vi "traces_free_find.vi"(0 "Thorlabs_OSA_64 in":refnum<class "OSA.lvclass">, 2 "idx start":i32, 4 "traces idx":cluster{"idx":u32}[](array[cluster]), 5 "error in (no error)":errorcluster, 6 "buffer size":i32, 7 "allocate X-array":bool) -> (14 "Thorlabs_OSA_64 out":refnum<class "OSA.lvclass">, 16 "idx found":i32, 18 "traces idx out":cluster{"idx":u32}[](array[cluster]), 19 "error out":errorcluster)   [LabVIEW 2010, in "OSA.lvclass"]
uses:
  OSA.lvclass
  FTSLib.dll
  OSA20X_misc.lvlib
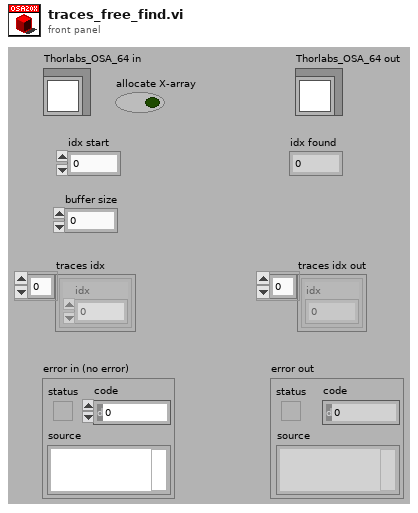
[diagram p1: front panel]
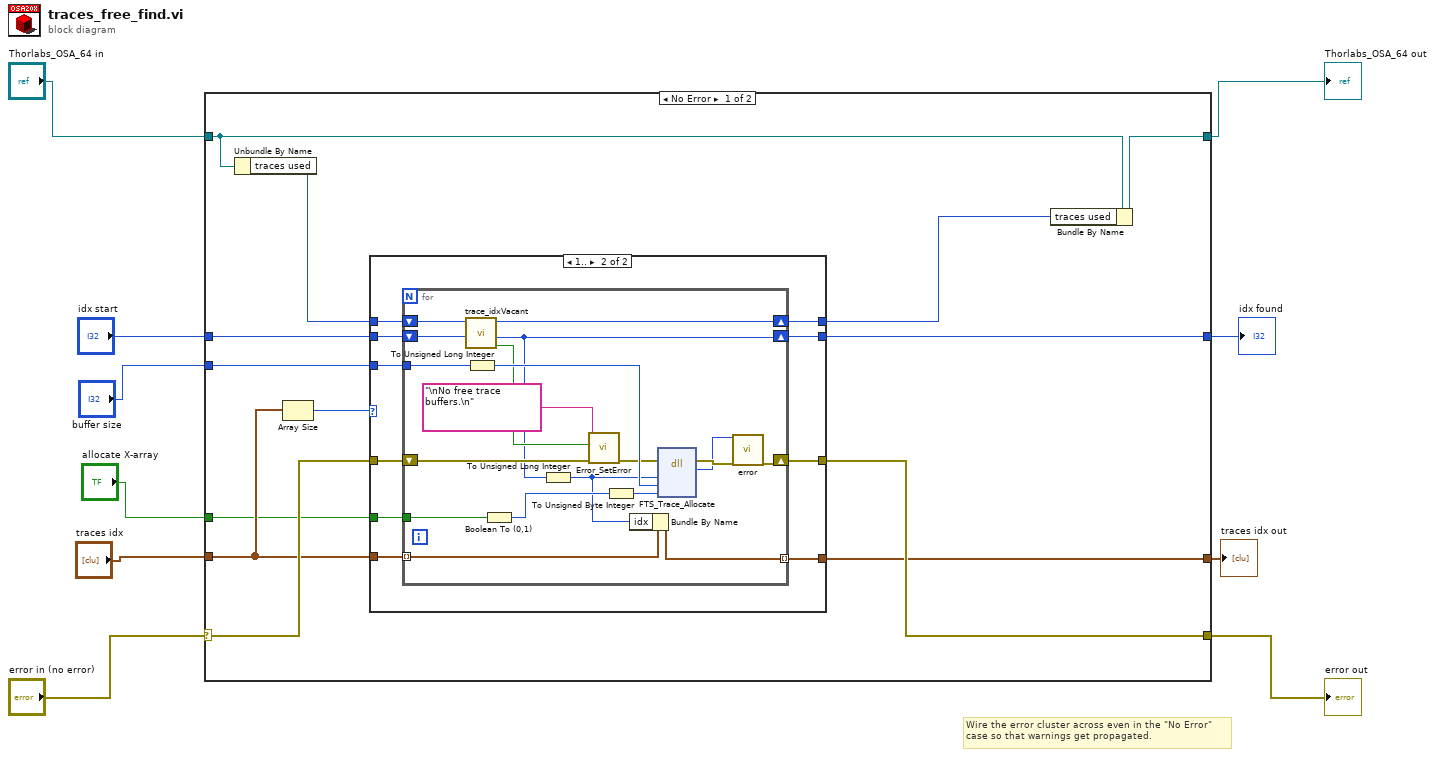
[diagram p0: block diagram]
diagram:
  # "Wire the error cluster across even in the \"No Error\"\ncase so that warnings get propagated."
  n1 = case shown="No Error" "error in (no error)" {
    selector: "error in (no error)" -> [w18 w60]
    tunnel: [w17 w60] -> w5
    tunnel: "idx start" -> [w20 w57]
    tunnel: [w19 w57] -> w9
    tunnel: "traces idx" -> [w16 w58]
    tunnel: [w15 w58] -> w7
    tunnel: "Thorlabs_OSA_64 in" -> [w14 w59]
    tunnel: [w13 w59] -> w3
    tunnel: "buffer size" -> [w12 _]
    tunnel: "allocate X-array" -> [w11 _]
    frame No Error {
      n2 = Unbundle By Name(w14) -> ("traces used"=w22:u64)
      n3 = Array Size(array=w16) -> (size(s)=w23:i32)
      n4 = case shown="1.." w23 {
        tunnel: w18 -> [w27 w37]
        tunnel: w12 -> [_ w36]
        tunnel: [w27 w35] -> w17
        tunnel: w16 -> [w26 w34]
        tunnel: [w26 w33] -> w15
        tunnel: w22 -> [w25 w32]
        tunnel: w20 -> [w24 w31]
        tunnel: [w25 w30] -> w21
        tunnel: [w24 w29] -> w19
        tunnel: w11 -> [_ w28]
        frame 0, Default {
        }
        frame 1.. {
          n5 = for {
            shift-right: [w53] -> w35
            shift-left: w37 -> [w44]
            tunnel: w36 -> [w56]
            tunnel: w34 -> [w51] mode=indexing
            tunnel: [w50] -> w33 mode=indexing
            shift-right: [w41] -> w30
            shift-left: w32 -> [w46]
            shift-right: [w39] -> w29
            shift-left: w31 -> [w45]
            tunnel: w28 -> [w38]
            n6 = call "trace_idxVacant.vi"("idx start"=w45, "traces active"=w46) -> ("none free"=w40:bool, "idx free"=w39:i32, "traces active out"=w41:u64)  [unwired: 7 in]
            n7 = To Unsigned Long Integer(number=w56) -> (unsigned 32bit integer=w55:u32)
            n8 = Boolean To (0,1)(Boolean=w38) -> (0, 1=w49:i16)
            n9 = To Unsigned Long Integer(number=w39) -> (unsigned 32bit integer=w47:u32)
            n10 = call "Error_SetError.vi"("error in"=w44, "status (true)"=w40, "source(\"\")"="\nNo free trace buffers.\n" ("source(\"\")")) -> ("error out"=w43:errorcluster)  [unwired: 4 in]
            n11 = To Unsigned Byte Integer(number=w49) -> (unsigned 8bit integer=w48:u8)
            n12 = Bundle By Name(cluster=w51, "idx"=w47) -> (w50:cluster{"idx":u32})
            n13 = dll-call lib="FTSLib.dll" fn="FTS_Trace_Allocate"(error in=w43, "idx_buffer"=w47, "length_data"=w55, "x_array"=w48) -> (error out=w54:errorcluster, "return type"=w52:i32)  [unwired: 5 in, 1 out]
            n14 = call "error.vi"("result code"=w52, "error in (no error)"=w54) -> ("error out"=w53:errorcluster)  [unwired: 15 in, 2 out]
          }
        }
      }
      n15 = Bundle By Name(cluster=w14, "traces used"=w21) -> (w13:refnum<class "OSA.lvclass">)
    }
    frame Error {
    }
  }
  "error out" <- w5
  "Thorlabs_OSA_64 out" <- w3
  "idx found" <- w9
  "traces idx out" <- w7
